vi "S4GUI.vi"() -> ()   [LabVIEW 2018] (continued)
            n1096 = call-dynamic "Write sequencia_ant.vi"("error in (no error)"=w2439, "sequencia_ant"=w2440, "Opt_Selector in"=w2442) -> ("error out"=w2438:errorcluster, "Opt_Selector out"=w2441:refnum<class "Opt_Selector.lvclass">)  [unwired: 7 in]
            n1097 = local write "P8"(w2447) -> ()
            n1098 = local write "P9"(w2447) -> ()
            n1099 = local write "P10"(w2447) -> ()
            n1100 = local write "P11"(w2447) -> ()
            n1101 = local write "P12"(w2445) -> ()
            n1102 = local write "P13"(w2445) -> ()
            n1103 = local write "P14"(w2445) -> ()
            n1104 = local write "P15"(w2445) -> ()
          }
          frame 1 {
            w2451 = u16 255 ("sequencia")
            w2458 = FALSE ("P0")
            w2459 = TRUE ("P0")
            w2460 = FALSE ("P0")
            w2461 = TRUE ("P0")
            # "0000 0000 1111 1111 = 255"
            n1105 = local write "P0"(w2461) -> ()
            n1106 = local write "P1"(w2461) -> ()
            n1107 = local write "P2"(w2461) -> ()
            n1108 = local write "P3"(w2461) -> ()
            n1109 = local write "P4"(w2459) -> ()
            n1110 = local write "P5"(w2459) -> ()
            n1111 = local write "P6"(w2459) -> ()
            n1112 = local write "P7"(w2459) -> ()
            n1113 = call-dynamic "Write sequencia.vi"("error in (no error)"=w2456, "sequencia"=w2451, "Opt_Selector in"=w2457) -> ("error out"=w2453:errorcluster, "Opt_Selector out"=w2455:refnum<class "Opt_Selector.lvclass">)  [unwired: 7 in]
            n1114 = local write "P8"(w2460) -> ()
            n1115 = local write "P9"(w2460) -> ()
            n1116 = local write "P10"(w2460) -> ()
            n1117 = local write "P11"(w2460) -> ()
            n1118 = local write "P12"(w2458) -> ()
            n1119 = local write "P13"(w2458) -> ()
            n1120 = local write "P14"(w2458) -> ()
            n1121 = local write "P15"(w2458) -> ()
            n1122 = call-dynamic "Write sequencia_ant.vi"("error in (no error)"=w2453, "sequencia_ant"=w2451, "Opt_Selector in"=w2455) -> ("error out"=w2452:errorcluster, "Opt_Selector out"=w2454:refnum<class "Opt_Selector.lvclass">)  [unwired: 7 in]
          }
          frame 2 {
            w2464 = u16 15 ("sequencia")
            w2471 = FALSE ("P0")
            w2472 = FALSE ("P0")
            w2473 = FALSE ("P0")
            w2474 = TRUE ("P0")
            # "0000 0000 0000 1111 = 15"
            n1123 = local write "P0"(w2474) -> ()
            n1124 = local write "P1"(w2474) -> ()
            n1125 = local write "P2"(w2474) -> ()
            n1126 = local write "P3"(w2474) -> ()
            n1127 = local write "P4"(w2472) -> ()
            n1128 = local write "P5"(w2472) -> ()
            n1129 = local write "P6"(w2472) -> ()
            n1130 = local write "P7"(w2472) -> ()
            n1131 = call-dynamic "Write sequencia.vi"("error in (no error)"=w2469, "sequencia"=w2464, "Opt_Selector in"=w2470) -> ("error out"=w2466:errorcluster, "Opt_Selector out"=w2468:refnum<class "Opt_Selector.lvclass">)  [unwired: 7 in]
            n1132 = call-dynamic "Write sequencia_ant.vi"("error in (no error)"=w2466, "sequencia_ant"=w2464, "Opt_Selector in"=w2468) -> ("error out"=w2465:errorcluster, "Opt_Selector out"=w2467:refnum<class "Opt_Selector.lvclass">)  [unwired: 7 in]
            n1133 = local write "P8"(w2473) -> ()
            n1134 = local write "P9"(w2473) -> ()
            n1135 = local write "P10"(w2473) -> ()
            n1136 = local write "P11"(w2473) -> ()
            n1137 = local write "P12"(w2471) -> ()
            n1138 = local write "P13"(w2471) -> ()
            n1139 = local write "P14"(w2471) -> ()
            n1140 = local write "P15"(w2471) -> ()
          }
          frame 3 {
            w2478 = u16 3855 ("sequencia")
            w2484 = FALSE ("P0")
            w2485 = FALSE ("P0")
            w2486 = TRUE ("P0")
            w2487 = TRUE ("P0")
            # "0000 1111 0000 1111 = 3855"
            n1141 = local write "P0"(w2487) -> ()
            n1142 = local write "P1"(w2487) -> ()
            n1143 = local write "P2"(w2487) -> ()
            n1144 = local write "P3"(w2487) -> ()
            n1145 = local write "P4"(w2485) -> ()
            n1146 = local write "P5"(w2485) -> ()
            n1147 = local write "P6"(w2485) -> ()
            n1148 = local write "P7"(w2485) -> ()
            n1149 = call-dynamic "Write sequencia.vi"("error in (no error)"=w2482, "sequencia"=w2478, "Opt_Selector in"=w2483) -> ("error out"=w2480:errorcluster, "Opt_Selector out"=w2481:refnum<class "Opt_Selector.lvclass">)  [unwired: 7 in]
            n1150 = local write "P8"(w2486) -> ()
            n1151 = local write "P9"(w2486) -> ()
            n1152 = local write "P10"(w2486) -> ()
            n1153 = local write "P11"(w2486) -> ()
            n1154 = local write "P12"(w2484) -> ()
            n1155 = local write "P13"(w2484) -> ()
            n1156 = local write "P14"(w2484) -> ()
            n1157 = local write "P15"(w2484) -> ()
            n1158 = call-dynamic "Write sequencia_ant.vi"("error in (no error)"=w2480, "sequencia_ant"=w2478, "Opt_Selector in"=w2481) -> ("error out"=w2479:errorcluster, "Opt_Selector out"=w2477:refnum<class "Opt_Selector.lvclass">)  [unwired: 7 in]
          }
          frame 4 {
            w2490 = u16 0 ("sequencia")
            w2497 = FALSE ("P0")
            w2498 = FALSE ("P0")
            w2499 = FALSE ("P0")
            w2500 = FALSE ("P0")
            n1159 = local write "P0"(w2500) -> ()
            n1160 = local write "P1"(w2500) -> ()
            n1161 = local write "P2"(w2500) -> ()
            n1162 = local write "P3"(w2500) -> ()
            n1163 = local write "P4"(w2498) -> ()
            n1164 = local write "P5"(w2498) -> ()
            n1165 = local write "P6"(w2498) -> ()
            n1166 = local write "P7"(w2498) -> ()
            n1167 = call-dynamic "Write sequencia.vi"("error in (no error)"=w2495, "sequencia"=w2490, "Opt_Selector in"=w2496) -> ("error out"=w2492:errorcluster, "Opt_Selector out"=w2494:refnum<class "Opt_Selector.lvclass">)  [unwired: 7 in]
            n1168 = call-dynamic "Write sequencia_ant.vi"("error in (no error)"=w2492, "sequencia_ant"=w2490, "Opt_Selector in"=w2494) -> ("error out"=w2491:errorcluster, "Opt_Selector out"=w2493:refnum<class "Opt_Selector.lvclass">)  [unwired: 7 in]
            n1169 = local write "P8"(w2499) -> ()
            n1170 = local write "P9"(w2499) -> ()
            n1171 = local write "P10"(w2499) -> ()
            n1172 = local write "P11"(w2499) -> ()
            n1173 = local write "P12"(w2497) -> ()
            n1174 = local write "P13"(w2497) -> ()
            n1175 = local write "P14"(w2497) -> ()
            n1176 = local write "P15"(w2497) -> ()
          }
          frame 5 {
          }
        }
        n1177 = call "Write WPROT.vi"("error in (no error)"=w2397, "Opt_Selector.lvclass"=w2404, "Instrument in"=w2403) -> ("error out"=w2406:errorcluster, "Instrument out"=w2407:refnum<class "Instrument.lvclass">)  [unwired: 7 in]
        n1178 = property on="#Polarimetric Sequence Done" class="Slide (strict)"(error in=w2397, "Scale.Maximum"=w2398, "Scale.Minimum"=w2396) -> ()  [unwired: 1 in, 2 out]
        n1179 = call "Write Instrument.lvclass.vi"("error in (no error)"=w2406, "Instrument.lvclass"=w2407, "S4ACS_GUI in"=w2402) -> ("error out"=w2386:errorcluster, "S4ACS_GUI out"=w2387:refnum<class "S4GUI.lvclass">)  [unwired: 7 in]
        n1180 = call "Read Instrument.lvclass.vi"("error in (no error)"=w2386, "S4ACS_GUI in"=w2387) -> ("error out"=w2391:errorcluster, "Instrument.lvclass"=w2392:refnum<class "Instrument.lvclass">, "S4ACS_GUI out"=w2395:refnum<class "S4GUI.lvclass">)  [unwired: 7 in]
        n1181 = call "Read ASEL.vi"("error in (no error)"=w2391, "Instrument in"=w2392) -> ("error out"=w2381:errorcluster, "Opt_Selector.lvclass"=w2383:refnum<class "Opt_Selector.lvclass">, "Instrument out"=w2388:refnum<class "Instrument.lvclass">)  [unwired: 7 in]
        n1182 = call "Read name_pos.vi"("error in (no error)"=w2381, "Optics in"=w2383) -> ("error out"=w2380:errorcluster, "name_pos"=w2379:string, "Optics out"=w2382:refnum<class "Opt_Selector.lvclass">)  [unwired: 7 in]
        n1183 = call "Write ASEL.vi"("error in (no error)"=w2380, "Opt_Selector.lvclass"=w2382, "Instrument in"=w2388) -> ("error out"=w2389:errorcluster, "Instrument out"=w2393:refnum<class "Instrument.lvclass">)  [unwired: 7 in]
        n1184 = case shown="\"ON\"" w2379 {
          tunnel: w2389 -> [w2412 w2423]
          tunnel: [w2412 w2419] -> w2390
          tunnel: w2393 -> [w2411 w2424]
          tunnel: [w2411 w2420] -> w2394
          frame Default {
          }
          frame "ON" {
            n1185 = call "Read WPROT.vi"("error in (no error)"=w2423, "Instrument in"=w2424) -> ("error out"=w2415:errorcluster, "Opt_Selector.lvclass"=w2422:refnum<class "Opt_Selector.lvclass">, "Instrument out"=w2421:refnum<class "Instrument.lvclass">)  [unwired: 7 in]
            n1186 = call-dynamic "Read sequencia.vi"("error in (no error)"=w2415, "Opt_Selector in"=w2422) -> ("error out"=w2414:errorcluster, "sequencia"=w2418:u16, "Opt_Selector out"=w2417:refnum<class "Opt_Selector.lvclass">)  [unwired: 7 in]
            n1187 = case shown="0" w2418 {
              tunnel: w2417 -> [w2426 w2435]
              tunnel: [w2426 w2431] -> w2416
              tunnel: w2414 -> [w2425 w2434]
              tunnel: [w2425 w2429] -> w2413
              frame Default {
              }
              frame 0 {
                n1188 = call-dynamic "Write sequencia.vi"("error in (no error)"=w2434, "sequencia"=u16 1, "Opt_Selector in"=w2435) -> ("error out"=w2430:errorcluster, "Opt_Selector out"=w2432:refnum<class "Opt_Selector.lvclass">)  [unwired: 7 in]
                n1189 = local write "P0"(TRUE ("P0")) -> ()
                n1190 = call-dynamic "Write sequencia_ant.vi"("error in (no error)"=w2430, "sequencia_ant"=u16 1, "Opt_Selector in"=w2432) -> ("error out"=w2429:errorcluster, "Opt_Selector out"=w2431:refnum<class "Opt_Selector.lvclass">)  [unwired: 7 in]
              }
            }
            n1191 = call "Write WPROT.vi"("error in (no error)"=w2413, "Opt_Selector.lvclass"=w2416, "Instrument in"=w2421) -> ("error out"=w2419:errorcluster, "Instrument out"=w2420:refnum<class "Instrument.lvclass">)  [unwired: 7 in]
          }
        }
        n1192 = call "Write Instrument.lvclass.vi"("error in (no error)"=w2390, "Instrument.lvclass"=w2394, "S4ACS_GUI in"=w2395) -> ("error out"=w2385:errorcluster, "S4ACS_GUI out"=w2384:refnum<class "S4GUI.lvclass">)  [unwired: 7 in]
      }
      event "P0", "P1", "P2", "P3", "P4", "P5", "P6", "P7", "P8", "P9", "P10", "P11", "P12", "P13", "P14", "P15": Value Change {
        w2558 = u16 5 items=["All 16 positions", "First 8 positions", "First 4 positions", "0-3 + 8-11", "Clear", "Customized"] ("Select Positions")
        # "Garantir que, quando em POLARIMETRIA, pelo menos WP1 esteja selecionado."
        # "Salva tambem em \nSequencia_ant para\no caso de repeticao."
        n1193 = event-data() -> ()  [unwired: 1 in, 6 out]
        n1194 = local write "Select Positions"(w2558) -> ()
        n1195 = call "Read Instrument.lvclass.vi"("error in (no error)"=w2540, "S4ACS_GUI in"=w2541) -> ("error out"=w2535:errorcluster, "Instrument.lvclass"=w2538:refnum<class "Instrument.lvclass">, "S4ACS_GUI out"=w2539:refnum<class "S4GUI.lvclass">)  [unwired: 7 in]
        n1196 = Build Array("P0", "P1", "P2", "P3", "P4", "P5", "P6", "P7", "P8", "P9", "P10", "P11", "P12", "P13", "P14", "P15") -> (w2526:bool[])
        n1197 = call "Read WPROT.vi"("error in (no error)"=w2535, "Instrument in"=w2538) -> ("error out"=w2534:errorcluster, "Opt_Selector.lvclass"=w2536:refnum<class "Opt_Selector.lvclass">, "Instrument out"=w2537:refnum<class "Instrument.lvclass">)  [unwired: 7 in]
        n1198 = Boolean Array To Number(Boolean array=w2526) -> (number=w2542:u32)
        n1199 = To Unsigned Word Integer(number=w2542) -> (unsigned 16bit integer=w2527:u16)
        n1200 = call-dynamic "Write sequencia.vi"("error in (no error)"=w2534, "sequencia"=w2527, "Opt_Selector in"=w2536) -> ("error out"=w2529:errorcluster, "Opt_Selector out"=w2531:refnum<class "Opt_Selector.lvclass">)  [unwired: 7 in]
        n1201 = call-dynamic "Write sequencia_ant.vi"("error in (no error)"=w2529, "sequencia_ant"=w2527, "Opt_Selector in"=w2531) -> ("error out"=w2528:errorcluster, "Opt_Selector out"=w2530:refnum<class "Opt_Selector.lvclass">)  [unwired: 7 in]
        n1202 = for {
          tunnel: w2526 -> [w2587] mode=indexing
          shift-right: [w2586] -> w2524
          shift-left: 0 -> [w2584]
          # "calcula qtd de 1s"
          n1203 = Increment(x=w2584) -> (x+1=w2585:i32)
          n1204 = Select(t=w2585, s=w2587, f=w2584) -> (s? t:f=w2586:i32)
        }
        n1205 = call "Write WPROT.vi"("error in (no error)"=w2528, "Opt_Selector.lvclass"=w2530, "Instrument in"=w2537) -> ("error out"=w2533:errorcluster, "Instrument out"=w2532:refnum<class "Instrument.lvclass">)  [unwired: 7 in]
        n1206 = call "Write Instrument.lvclass.vi"("error in (no error)"=w2533, "Instrument.lvclass"=w2532, "S4ACS_GUI in"=w2539) -> ("error out"=w2507:errorcluster, "S4ACS_GUI out"=w2508:refnum<class "S4GUI.lvclass">)  [unwired: 7 in]
        n1207 = property on="#Polarimetric Sequence Done" class="Slide (strict)"("Scale.Maximum"=w2524, "Scale.Minimum"=0.0 ("Scale.Range:Minimum")) -> ()  [unwired: 2 in, 2 out]
        n1208 = call "Read Instrument.lvclass.vi"("error in (no error)"=w2507, "S4ACS_GUI in"=w2508) -> ("error out"=w2513:errorcluster, "Instrument.lvclass"=w2512:refnum<class "Instrument.lvclass">, "S4ACS_GUI out"=w2509:refnum<class "S4GUI.lvclass">)  [unwired: 7 in]
        n1209 = call "Read ASEL.vi"("error in (no error)"=w2513, "Instrument in"=w2512) -> ("error out"=w2519:errorcluster, "Opt_Selector.lvclass"=w2517:refnum<class "Opt_Selector.lvclass">, "Instrument out"=w2516:refnum<class "Instrument.lvclass">)  [unwired: 7 in]
        n1210 = call "Read name_pos.vi"("error in (no error)"=w2519, "Optics in"=w2517) -> ("error out"=w2520:errorcluster, "name_pos"=w2521:string, "Optics out"=w2518:refnum<class "Opt_Selector.lvclass">)  [unwired: 7 in]
        n1211 = call "Write ASEL.vi"("error in (no error)"=w2520, "Opt_Selector.lvclass"=w2518, "Instrument in"=w2516) -> ("error out"=w2515:errorcluster, "Instrument out"=w2511:refnum<class "Instrument.lvclass">)  [unwired: 7 in]
        n1212 = case shown="\"ON\"" w2521 {
          tunnel: w2515 -> [w2560 w2571]
          tunnel: [w2560 w2567] -> w2514
          tunnel: w2511 -> [w2559 w2572]
          tunnel: [w2559 w2568] -> w2510
          frame Default {
          }
          frame "ON" {
            n1213 = call "Read WPROT.vi"("error in (no error)"=w2571, "Instrument in"=w2572) -> ("error out"=w2563:errorcluster, "Opt_Selector.lvclass"=w2570:refnum<class "Opt_Selector.lvclass">, "Instrument out"=w2569:refnum<class "Instrument.lvclass">)  [unwired: 7 in]
            n1214 = call-dynamic "Read sequencia.vi"("error in (no error)"=w2563, "Opt_Selector in"=w2570) -> ("error out"=w2562:errorcluster, "sequencia"=w2566:u16, "Opt_Selector out"=w2565:refnum<class "Opt_Selector.lvclass">)  [unwired: 7 in]
            n1215 = case shown="0" w2566 {
              tunnel: w2565 -> [w2574 w2583]
              tunnel: [w2574 w2579] -> w2564
              tunnel: w2562 -> [w2573 w2582]
              tunnel: [w2573 w2577] -> w2561
              frame Default {
              }
              frame 0 {
                n1216 = call-dynamic "Write sequencia.vi"("error in (no error)"=w2582, "sequencia"=u16 1, "Opt_Selector in"=w2583) -> ("error out"=w2578:errorcluster, "Opt_Selector out"=w2580:refnum<class "Opt_Selector.lvclass">)  [unwired: 7 in]
                n1217 = local write "P0"(TRUE ("P0")) -> ()
                n1218 = call-dynamic "Write sequencia_ant.vi"("error in (no error)"=w2578, "sequencia_ant"=u16 1, "Opt_Selector in"=w2580) -> ("error out"=w2577:errorcluster, "Opt_Selector out"=w2579:refnum<class "Opt_Selector.lvclass">)  [unwired: 7 in]
              }
            }
            n1219 = call "Write WPROT.vi"("error in (no error)"=w2561, "Opt_Selector.lvclass"=w2564, "Instrument in"=w2569) -> ("error out"=w2567:errorcluster, "Instrument out"=w2568:refnum<class "Instrument.lvclass">)  [unwired: 7 in]
          }
        }
        n1220 = call "Write Instrument.lvclass.vi"("error in (no error)"=w2514, "Instrument.lvclass"=w2510, "S4ACS_GUI in"=w2509) -> ("error out"=w2505:errorcluster, "S4ACS_GUI out"=w2506:refnum<class "S4GUI.lvclass">)  [unwired: 7 in]
      }
      event "SSM": Value Change {
        # "F: fotom.\nT: polar."
        n1221 = event-data() -> ()  [unwired: 1 in, 6 out]
        n1222 = call-dynamic "Read mode EXPOSE.vi"("error in (no error)"=w2593, "S4GUI in"=w2594) -> ("error out"=w2592:errorcluster, "mode EXPOSE"=w2588:bool, "S4GUI out"=w2589:refnum<class "S4GUI.lvclass">)  [unwired: 7 in]
        n1223 = call "Read Instrument.lvclass.vi"("error in (no error)"=w2592, "S4ACS_GUI in"=w2589) -> ("error out"=w2591:errorcluster, "Instrument.lvclass"=w2597:refnum<class "Instrument.lvclass">, "S4ACS_GUI out"=w2596:refnum<class "S4GUI.lvclass">)  [unwired: 7 in]
        n1224 = call-dynamic "Read mode.vi"("error in (no error)"=w2591, "Instrument in"=w2597) -> ("error out"=w2590:errorcluster, "mode"=w2595:bool)  [unwired: 7 in, 1 out]
        n1225 = case shown="0, Default" "SSM" {
          tunnel: [T7."Enabled" ("Disabled") T7."Disabled and Grayed Out" ("Disabled")] -> w2630
          tunnel: [T7."Disabled and Grayed Out" ("Disabled") T7."Enabled" ("Disabled")] -> w2611
          tunnel: [w2646 "Start" ("Caption.Text")] -> w2622
          tunnel: [w2646 "Stop" ("Caption.Text")] -> w2615
          tunnel: [w2646 "Abort" ("Caption.Text")] -> w2610
          tunnel: [w2646 "Pause" ("Caption.Text")] -> w2617
          tunnel: [TRUE FALSE] -> w2628
          tunnel: [T7."Enabled" ("Disabled") T7."Disabled and Grayed Out" ("Disabled")] -> w2625
          tunnel: [T7."Disabled and Grayed Out" ("Disabled") T7."Enabled" ("Disabled")] -> w2605
          tunnel: w2590 -> [w2638 w2873]
          tunnel: w2596 -> [w2640 w2872]
          tunnel: [w2642 w2864] -> w2603
          tunnel: [w2634 w2863] -> w2602
          tunnel: w2595 -> [_ w2849]
          tunnel: w2588 -> [_ w2847]
          frame 1 {
            w2646 = "Sync" ("Caption.Text")
            # "Sync mode: Os canais sao configurados para Trigger externo, desde que o SyncBox esteja conectado."
            # "Sync by Cycle"
            n1226 = call-dynamic "Read Sync Box.lvclass.vi"("error in (no error)"=w2638, "SPARC4_AC in"=w2640) -> ("error out"=w2637:errorcluster, "Sync Box.lvclass"=w2641:refnum<class "Sync Box.lvclass">, "SPARC4_AC out"=w2639:refnum<class "S4GUI.lvclass">)  [unwired: 7 in]
            n1227 = call "Read connection.vi"("error in (no error)"=w2637, "Server in"=w2641) -> ("error out"=w2636:errorcluster, "connection"=w2635:bool)  [unwired: 7 in, 1 out]
            n1228 = case shown="True" w2635 {
              tunnel: [w2650 w2667] -> w2642
              tunnel: w2639 -> [w2650 w2657]
              tunnel: w2636 -> [w2649 w2656]
              tunnel: [w2649 w2651] -> w2634
              frame False {
              }
              frame True {
                n1229 = call-dynamic "Read AcquisitionC.vi"("error in (no error)"=w2656, "S4ACS_GUI in"=w2657) -> ("error out"=w2674:errorcluster, "Acquisition.lvclass"=w2673:refnum<class "Acquisition.lvclass">)  [unwired: 7 in, 1 out]
                n1230 = call-dynamic "Read AcquisitionA.vi"("error in (no error)"=w2656, "S4ACS_GUI in"=w2657) -> ("error out"=w2677:errorcluster, "Acquisition.lvclass"=w2678:refnum<class "Acquisition.lvclass">, "S4ACS_GUI out"=w2666:refnum<class "S4GUI.lvclass">)  [unwired: 7 in]
                n1231 = call "Read AcquisitionB.vi"("error in (no error)"=w2656, "S4ACS_GUI in"=w2657) -> ("error out"=w2675:errorcluster, "Acquisition.lvclass"=w2676:refnum<class "Acquisition.lvclass">)  [unwired: 7 in, 1 out]
                n1232 = call-dynamic "Read AcquisitionD.vi"("error in (no error)"=w2656, "S4ACS_GUI in"=w2657) -> ("error out"=w2671:errorcluster, "Acquisition.lvclass"=w2672:refnum<class "Acquisition.lvclass">)  [unwired: 7 in, 1 out]
                n1233 = call "Read connection.vi"("error in (no error)"=w2671, "Server in"=w2672) -> ("error out"=w2680:errorcluster, "connection"=w2679:bool, "Server out"=w2681:refnum<class "Acquisition.lvclass">)  [unwired: 7 in]
                n1234 = call "Read connection.vi"("error in (no error)"=w2674, "Server in"=w2673) -> ("error out"=w2683:errorcluster, "connection"=w2682:bool, "Server out"=w2684:refnum<class "Acquisition.lvclass">)  [unwired: 7 in]
                n1235 = call "Read connection.vi"("error in (no error)"=w2675, "Server in"=w2676) -> ("error out"=w2686:errorcluster, "connection"=w2685:bool, "Server out"=w2687:refnum<class "Acquisition.lvclass">)  [unwired: 7 in]
                n1236 = call "Read connection.vi"("error in (no error)"=w2677, "Server in"=w2678) -> ("error out"=w2689:errorcluster, "connection"=w2688:bool, "Server out"=w2690:refnum<class "Acquisition.lvclass">)  [unwired: 7 in]
                n1237 = case shown="True" w2685 {
                  tunnel: w2687 -> [w2770 w2774]
                  tunnel: w2686 -> [w2769 w2773]
                  tunnel: [w2770 w2772] -> w2663
                  tunnel: [w2769 w2771] -> w2662
                  frame False {
                  }
                  frame True {
                    # "Ext Start"
                    # "nome do arquivo .cfg"
                    # "seção no arquivo .cfg"
                    n1238 = call-dynamic "Read Channel.vi"("error in (no error)"=w2773, "Acquisition in"=w2774) -> ("error out"=w2778:errorcluster, "Channel.lvclass"=w2777:refnum<class "Channel.lvclass">, "Acquisition out"=w2776:refnum<class "Acquisition.lvclass">)  [unwired: 7 in]
                    n1239 = call-dynamic "Read Interface.vi"("error in (no error)"=w2778, "Channel in"=w2777) -> ("error out"=w2786:errorcluster, "Interface.lvclass"=w2787:refnum<class "Interface.lvclass">, "Channel out"=w2775:refnum<class "Channel.lvclass">)  [unwired: 7 in]
                    n1240 = call-dynamic "Get CCD_Config.vi"("error in (no error)"=w2786, "Interface in"=w2787) -> ("error out"=w2783:errorcluster, "output cluster"=w2782:T24, "Interface out"=w2788:refnum<class "Interface.lvclass">)  [unwired: 7 in]
                    n1241 = Bundle By Name(cluster=w2782, "TRIGGER_MODE"=u8 6 ("SHUTTER_MODE")) -> (w2784:T24)
                    n1242 = call-dynamic "Set CCD_Config.vi"("error in (no error)"=w2783, "input cluster"=w2784, "Interface in"=w2788) -> ("error out"=w2781:errorcluster, "Interface out"=w2789:refnum<class "Interface.lvclass">)  [unwired: 7 in]
                    n1243 = Flatten To String(anything=w2784, error in (no error)=w2781) -> (data string=w2779:string, error out=w2780:errorcluster)  [unwired: 2 in, 1 out]
                    n1244 = call "Write flatted cluster.vi"("error in (no error)"=w2780, "flatted cluster"=w2779, "Interface in"=w2789) -> ("error out"=w2791:errorcluster, "Interface out"=w2790:refnum<class "Interface.lvclass">)  [unwired: 7 in]
                    n1245 = call-dynamic "Write Interface.vi"("error in (no error)"=w2791, "Interface.lvclass"=w2790, "Channel in"=w2775) -> ("error out"=w2797:errorcluster, "Channel out"=w2798:refnum<class "Channel.lvclass">)  [unwired: 7 in]
                    n1246 = call "Write section_name.vi"("error in (no error)"=w2797, "section_name"="CCD_ACS2", "Channel in"=w2798) -> ("error out"=w2795:errorcluster, "Channel out"=w2801:refnum<class "Channel.lvclass">)  [unwired: 7 in]
                    n1247 = call-dynamic "save config.vi"("error in (no error)"=w2795, "file config"="lastsaved.cfg", "Channel in"=w2801) -> ("error out"=w2796:errorcluster, "Channel out"=w2802:refnum<class "Channel.lvclass">)  [unwired: 7 in]
                    n1248 = call-dynamic "Read State Machine.vi"("error in (no error)"=w2796, "Device in"=w2802) -> ("error out"=w2792:errorcluster, "State Machine.lvclass"=w2804:refnum<class "State Machine.lvclass">, "Device out"=w2803:refnum<class "Channel.lvclass">)  [unwired: 7 in]
                    n1249 = call-dynamic "Write State.vi"("error in (no error)"=w2792, "State"=60, "State Machine in"=w2804) -> ("error out"=w2793:errorcluster, "State Machine out"=w2805:refnum<class "State Machine.lvclass">)  [unwired: 7 in]
                    n1250 = call-dynamic "Write State Machine.vi"("error in (no error)"=w2793, "State Machine.lvclass"=w2805, "Device in"=w2803) -> ("error out"=w2807:errorcluster, "Device out"=w2806:refnum<class "Channel.lvclass">)  [unwired: 7 in]
                    n1251 = call-dynamic "Write Channel.vi"("error in (no error)"=w2807, "Channel.lvclass"=w2806, "Acquisition in"=w2776) -> ("error out"=w2771:errorcluster, "Acquisition out"=w2772:refnum<class "Acquisition.lvclass">)  [unwired: 7 in]
                  }
                }
                n1252 = case shown="True" w2688 {
                  tunnel: [w2808 w2842] -> w2664
                  tunnel: [w2809 w2841] -> w2665
                  tunnel: w2690 -> [w2809 w2811]
                  tunnel: w2689 -> [w2808 w2810]
                  frame False {
                  }
                  frame True {
                    # "nome do arquivo .cfg"
                    # "seção no arquivo .cfg"
                    # "Ext Start"
                    n1253 = call-dynamic "Read Channel.vi"("error in (no error)"=w2810, "Acquisition in"=w2811) -> ("error out"=w2843:errorcluster, "Channel.lvclass"=w2844:refnum<class "Channel.lvclass">, "Acquisition out"=w2845:refnum<class "Acquisition.lvclass">)  [unwired: 7 in]
                    n1254 = call-dynamic "Read Interface.vi"("error in (no error)"=w2843, "Channel in"=w2844) -> ("error out"=w2833:errorcluster, "Interface.lvclass"=w2832:refnum<class "Interface.lvclass">, "Channel out"=w2846:refnum<class "Channel.lvclass">)  [unwired: 7 in]
                    n1255 = call-dynamic "Get CCD_Config.vi"("error in (no error)"=w2833, "Interface in"=w2832) -> ("error out"=w2836:errorcluster, "output cluster"=w2837:T24, "Interface out"=w2831:refnum<class "Interface.lvclass">)  [unwired: 7 in]
                    n1256 = Bundle By Name(cluster=w2837, "TRIGGER_MODE"=u8 6 ("SHUTTER_MODE")) -> (w2835:T24)
                    n1257 = call-dynamic "Set CCD_Config.vi"("error in (no error)"=w2836, "input cluster"=w2835, "Interface in"=w2831) -> ("error out"=w2838:errorcluster, "Interface out"=w2830:refnum<class "Interface.lvclass">)  [unwired: 7 in]
                    n1258 = Flatten To String(anything=w2835, error in (no error)=w2838) -> (data string=w2840:string, error out=w2839:errorcluster)  [unwired: 2 in, 1 out]
                    n1259 = call "Write flatted cluster.vi"("error in (no error)"=w2839, "flatted cluster"=w2840, "Interface in"=w2830) -> ("error out"=w2828:errorcluster, "Interface out"=w2829:refnum<class "Interface.lvclass">)  [unwired: 7 in]
                    n1260 = call-dynamic "Write Interface.vi"("error in (no error)"=w2828, "Interface.lvclass"=w2829, "Channel in"=w2846) -> ("error out"=w2823:errorcluster, "Channel out"=w2822:refnum<class "Channel.lvclass">)  [unwired: 7 in]
                    n1261 = call "Write section_name.vi"("error in (no error)"=w2823, "section_name"="CCD_ACS1", "Channel in"=w2822) -> ("error out"=w2824:errorcluster, "Channel out"=w2819:refnum<class "Channel.lvclass">)  [unwired: 7 in]
                    n1262 = call-dynamic "save config.vi"("error in (no error)"=w2824, "file config"="lastsaved.cfg", "Channel in"=w2819) -> ("error out"=w2812:errorcluster, "Channel out"=w2813:refnum<class "Channel.lvclass">)  [unwired: 7 in]
                    n1263 = call-dynamic "Read State Machine.vi"("error in (no error)"=w2812, "Device in"=w2813) -> ("error out"=w2827:errorcluster, "State Machine.lvclass"=w2817:refnum<class "State Machine.lvclass">, "Device out"=w2818:refnum<class "Channel.lvclass">)  [unwired: 7 in]
                    n1264 = call-dynamic "Write State.vi"("error in (no error)"=w2827, "State"=60, "State Machine in"=w2817) -> ("error out"=w2826:errorcluster, "State Machine out"=w2816:refnum<class "State Machine.lvclass">)  [unwired: 7 in]
                    n1265 = call-dynamic "Write State Machine.vi"("error in (no error)"=w2826, "State Machine.lvclass"=w2816, "Device in"=w2818) -> ("error out"=w2814:errorcluster, "Device out"=w2815:refnum<class "Channel.lvclass">)  [unwired: 7 in]
                    n1266 = call-dynamic "Write Channel.vi"("error in (no error)"=w2814, "Channel.lvclass"=w2815, "Acquisition in"=w2845) -> ("error out"=w2842:errorcluster, "Acquisition out"=w2841:refnum<class "Acquisition.lvclass">)  [unwired: 7 in]
                  }
                }
                n1267 = case shown="True" w2682 {
                  tunnel: w2684 -> [w2731 w2735]
                  tunnel: w2683 -> [w2730 w2734]
                  tunnel: [w2731 w2733] -> w2661
                  tunnel: [w2730 w2732] -> w2660
                  frame False {
                  }
                  frame True {
                    # "Ext Start"
                    # "nome do arquivo .cfg"
                    # "seção no arquivo .cfg"
                    n1268 = call-dynamic "Read Channel.vi"("error in (no error)"=w2734, "Acquisition in"=w2735) -> ("error out"=w2739:errorcluster, "Channel.lvclass"=w2738:refnum<class "Channel.lvclass">, "Acquisition out"=w2737:refnum<class "Acquisition.lvclass">)  [unwired: 7 in]
                    n1269 = call-dynamic "Read Interface.vi"("error in (no error)"=w2739, "Channel in"=w2738) -> ("error out"=w2747:errorcluster, "Interface.lvclass"=w2748:refnum<class "Interface.lvclass">, "Channel out"=w2736:refnum<class "Channel.lvclass">)  [unwired: 7 in]
                    n1270 = call-dynamic "Get CCD_Config.vi"("error in (no error)"=w2747, "Interface in"=w2748) -> ("error out"=w2744:errorcluster, "output cluster"=w2743:T24, "Interface out"=w2749:refnum<class "Interface.lvclass">)  [unwired: 7 in]
                    n1271 = Bundle By Name(cluster=w2743, "TRIGGER_MODE"=u8 6 ("SHUTTER_MODE")) -> (w2745:T24)
                    n1272 = call-dynamic "Set CCD_Config.vi"("error in (no error)"=w2744, "input cluster"=w2745, "Interface in"=w2749) -> ("error out"=w2742:errorcluster, "Interface out"=w2750:refnum<class "Interface.lvclass">)  [unwired: 7 in]
                    n1273 = Flatten To String(anything=w2745, error in (no error)=w2742) -> (data string=w2740:string, error out=w2741:errorcluster)  [unwired: 2 in, 1 out]
                    n1274 = call "Write flatted cluster.vi"("error in (no error)"=w2741, "flatted cluster"=w2740, "Interface in"=w2750) -> ("error out"=w2752:errorcluster, "Interface out"=w2751:refnum<class "Interface.lvclass">)  [unwired: 7 in]
                    n1275 = call-dynamic "Write Interface.vi"("error in (no error)"=w2752, "Interface.lvclass"=w2751, "Channel in"=w2736) -> ("error out"=w2758:errorcluster, "Channel out"=w2759:refnum<class "Channel.lvclass">)  [unwired: 7 in]
                    n1276 = call "Write section_name.vi"("error in (no error)"=w2758, "section_name"="CCD_ACS3", "Channel in"=w2759) -> ("error out"=w2756:errorcluster, "Channel out"=w2762:refnum<class "Channel.lvclass">)  [unwired: 7 in]
                    n1277 = call-dynamic "save config.vi"("error in (no error)"=w2756, "file config"="lastsaved.cfg", "Channel in"=w2762) -> ("error out"=w2757:errorcluster, "Channel out"=w2763:refnum<class "Channel.lvclass">)  [unwired: 7 in]
                    n1278 = call-dynamic "Read State Machine.vi"("error in (no error)"=w2757, "Device in"=w2763) -> ("error out"=w2753:errorcluster, "State Machine.lvclass"=w2765:refnum<class "State Machine.lvclass">, "Device out"=w2764:refnum<class "Channel.lvclass">)  [unwired: 7 in]
                    n1279 = call-dynamic "Write State.vi"("error in (no error)"=w2753, "State"=60, "State Machine in"=w2765) -> ("error out"=w2754:errorcluster, "State Machine out"=w2766:refnum<class "State Machine.lvclass">)  [unwired: 7 in]
                    n1280 = call-dynamic "Write State Machine.vi"("error in (no error)"=w2754, "State Machine.lvclass"=w2766, "Device in"=w2764) -> ("error out"=w2768:errorcluster, "Device out"=w2767:refnum<class "Channel.lvclass">)  [unwired: 7 in]
                    n1281 = call-dynamic "Write Channel.vi"("error in (no error)"=w2768, "Channel.lvclass"=w2767, "Acquisition in"=w2737) -> ("error out"=w2732:errorcluster, "Acquisition out"=w2733:refnum<class "Acquisition.lvclass">)  [unwired: 7 in]
                  }
                }
                n1282 = case shown="True" w2679 {
                  tunnel: w2681 -> [w2692 w2696]
                  tunnel: w2680 -> [w2691 w2695]
                  tunnel: [w2692 w2694] -> w2659
                  tunnel: [w2691 w2693] -> w2658
                  frame False {
                  }
                  frame True {
                    # "Ext Start"
                    # "nome do arquivo .cfg"
                    # "seção no arquivo .cfg"
                    n1283 = call-dynamic "Read Channel.vi"("error in (no error)"=w2695, "Acquisition in"=w2696) -> ("error out"=w2726:errorcluster, "Channel.lvclass"=w2727:refnum<class "Channel.lvclass">, "Acquisition out"=w2728:refnum<class "Acquisition.lvclass">)  [unwired: 7 in]
                    n1284 = call-dynamic "Read Interface.vi"("error in (no error)"=w2726, "Channel in"=w2727) -> ("error out"=w2718:errorcluster, "Interface.lvclass"=w2717:refnum<class "Interface.lvclass">, "Channel out"=w2729:refnum<class "Channel.lvclass">)  [unwired: 7 in]
                    n1285 = call-dynamic "Get CCD_Config.vi"("error in (no error)"=w2718, "Interface in"=w2717) -> ("error out"=w2721:errorcluster, "output cluster"=w2722:T24, "Interface out"=w2716:refnum<class "Interface.lvclass">)  [unwired: 7 in]
                    n1286 = Bundle By Name(cluster=w2722, "TRIGGER_MODE"=u8 6 ("SHUTTER_MODE")) -> (w2720:T24)
                    n1287 = call-dynamic "Set CCD_Config.vi"("error in (no error)"=w2721, "input cluster"=w2720, "Interface in"=w2716) -> ("error out"=w2723:errorcluster, "Interface out"=w2715:refnum<class "Interface.lvclass">)  [unwired: 7 in]
                    n1288 = Flatten To String(anything=w2720, error in (no error)=w2723) -> (data string=w2725:string, error out=w2724:errorcluster)  [unwired: 2 in, 1 out]
                    n1289 = call "Write flatted cluster.vi"("error in (no error)"=w2724, "flatted cluster"=w2725, "Interface in"=w2715) -> ("error out"=w2713:errorcluster, "Interface out"=w2714:refnum<class "Interface.lvclass">)  [unwired: 7 in]
                    n1290 = call-dynamic "Write Interface.vi"("error in (no error)"=w2713, "Interface.lvclass"=w2714, "Channel in"=w2729) -> ("error out"=w2707:errorcluster, "Channel out"=w2706:refnum<class "Channel.lvclass">)  [unwired: 7 in]
                    n1291 = call "Write section_name.vi"("error in (no error)"=w2707, "section_name"="CCD_ACS4", "Channel in"=w2706) -> ("error out"=w2709:errorcluster, "Channel out"=w2703:refnum<class "Channel.lvclass">)  [unwired: 7 in]
                    n1292 = call-dynamic "save config.vi"("error in (no error)"=w2709, "file config"="lastsaved.cfg", "Channel in"=w2703) -> ("error out"=w2708:errorcluster, "Channel out"=w2702:refnum<class "Channel.lvclass">)  [unwired: 7 in]
                    n1293 = call-dynamic "Read State Machine.vi"("error in (no error)"=w2708, "Device in"=w2702) -> ("error out"=w2712:errorcluster, "State Machine.lvclass"=w2700:refnum<class "State Machine.lvclass">, "Device out"=w2701:refnum<class "Channel.lvclass">)  [unwired: 7 in]
                    n1294 = call-dynamic "Write State.vi"("error in (no error)"=w2712, "State"=60, "State Machine in"=w2700) -> ("error out"=w2711:errorcluster, "State Machine out"=w2699:refnum<class "State Machine.lvclass">)  [unwired: 7 in]
                    n1295 = call-dynamic "Write State Machine.vi"("error in (no error)"=w2711, "State Machine.lvclass"=w2699, "Device in"=w2701) -> ("error out"=w2697:errorcluster, "Device out"=w2698:refnum<class "Channel.lvclass">)  [unwired: 7 in]
                    n1296 = call-dynamic "Write Channel.vi"("error in (no error)"=w2697, "Channel.lvclass"=w2698, "Acquisition in"=w2728) -> ("error out"=w2693:errorcluster, "Acquisition out"=w2694:refnum<class "Acquisition.lvclass">)  [unwired: 7 in]
                  }
                }
                n1297 = call-dynamic "Write AcquisitionA.vi"("error in (no error)"=w2664, "Acquisition.lvclass"=w2665, "S4ACS_GUI in"=w2666) -> ("error out"=w2655:errorcluster, "S4ACS_GUI out"=w2670:refnum<class "S4GUI.lvclass">)  [unwired: 7 in]
                n1298 = call "Write AcquisitionB.vi"("error in (no error)"=w2662, "Acquisition.lvclass"=w2663, "S4ACS_GUI in"=w2670) -> ("error out"=w2654:errorcluster, "S4ACS_GUI out"=w2669:refnum<class "S4GUI.lvclass">)  [unwired: 7 in]
                n1299 = call-dynamic "Write AcquisitionC.vi"("error in (no error)"=w2660, "Acquisition.lvclass"=w2661, "S4ACS_GUI in"=w2669) -> ("error out"=w2653:errorcluster, "S4ACS_GUI out"=w2668:refnum<class "S4GUI.lvclass">)  [unwired: 7 in]
                n1300 = call-dynamic "Write AcquisitionD.vi"("error in (no error)"=w2658, "Acquisition.lvclass"=w2659, "S4ACS_GUI in"=w2668) -> ("error out"=w2652:errorcluster, "S4ACS_GUI out"=w2667:refnum<class "S4GUI.lvclass">)  [unwired: 7 in]
                n1301 = Merge Errors(w2655, w2654, w2653, w2652) -> (w2651:errorcluster)
              }
            }
          }
          frame 0, Default {
            # "Async mode: Os canais são configurados com Trigger Interno para Fotometria ou Trigger Externo para Polarimetria (independentemente do status do SyncBox)"
            # "Aynchronous:"
            n1302 = call-dynamic "Read AcquisitionC.vi"("error in (no error)"=w2873, "S4ACS_GUI in"=w2872) -> ("error out"=w2877:errorcluster, "Acquisition.lvclass"=w2876:refnum<class "Acquisition.lvclass">)  [unwired: 7 in, 1 out]
            n1303 = call "Read AcquisitionB.vi"("error in (no error)"=w2873, "S4ACS_GUI in"=w2872) -> ("error out"=w2878:errorcluster, "Acquisition.lvclass"=w2879:refnum<class "Acquisition.lvclass">)  [unwired: 7 in, 1 out]
            n1304 = call-dynamic "Read AcquisitionA.vi"("error in (no error)"=w2873, "S4ACS_GUI in"=w2872) -> ("error out"=w2880:errorcluster, "Acquisition.lvclass"=w2881:refnum<class "Acquisition.lvclass">, "S4ACS_GUI out"=w2862:refnum<class "S4GUI.lvclass">)  [unwired: 7 in]
            n1305 = case shown="True" w2849 {
              tunnel: [u8 0 ("SHUTTER_MODE") w2900] -> w2848
              tunnel: w2847 -> [_ w2903]
              frame False {
                # "Fotom."
                # "Internal"
              }
              frame True {
                # "exp mode?"
                # "Internal"
                # "Polar."
                # "Ext. Start"
                n1306 = Select(t=u8 0, s=w2903, f=u8 6 ("SHUTTER_MODE")) -> (s? t:f=w2900:u8)
              }
            }
            n1307 = call-dynamic "Read AcquisitionD.vi"("error in (no error)"=w2873, "S4ACS_GUI in"=w2872) -> ("error out"=w2874:errorcluster, "Acquisition.lvclass"=w2875:refnum<class "Acquisition.lvclass">)  [unwired: 7 in, 1 out]
            n1308 = call "Read connection.vi"("error in (no error)"=w2877, "Server in"=w2876) -> ("error out"=w2886:errorcluster, "connection"=w2885:bool, "Server out"=w2887:refnum<class "Acquisition.lvclass">)  [unwired: 7 in]
            n1309 = call "Read connection.vi"("error in (no error)"=w2878, "Server in"=w2879) -> ("error out"=w2889:errorcluster, "connection"=w2888:bool, "Server out"=w2890:refnum<class "Acquisition.lvclass">)  [unwired: 7 in]
            n1310 = call "Read connection.vi"("error in (no error)"=w2874, "Server in"=w2875) -> ("error out"=w2883:errorcluster, "connection"=w2882:bool, "Server out"=w2884:refnum<class "Acquisition.lvclass">)  [unwired: 7 in]
            n1311 = call "Read connection.vi"("error in (no error)"=w2880, "Server in"=w2881) -> ("error out"=w2892:errorcluster, "connection"=w2891:bool, "Server out"=w2893:refnum<class "Acquisition.lvclass">)  [unwired: 7 in]
            n1312 = case shown="True" w2885 {
              tunnel: w2887 -> [w2944 w2949]
              tunnel: w2886 -> [w2943 w2948]
              tunnel: [w2944 w2947] -> w2857
              tunnel: [w2943 w2946] -> w2856
              tunnel: w2848 -> [_ w2945]
              frame False {
              }
              frame True {
                # "nome do arquivo .cfg"
                # "seção no arquivo .cfg"
                n1313 = call-dynamic "Read Channel.vi"("error in (no error)"=w2948, "Acquisition in"=w2949) -> ("error out"=w2953:errorcluster, "Channel.lvclass"=w2952:refnum<class "Channel.lvclass">, "Acquisition out"=w2951:refnum<class "Acquisition.lvclass">)  [unwired: 7 in]
                n1314 = call-dynamic "Read Interface.vi"("error in (no error)"=w2953, "Channel in"=w2952) -> ("error out"=w2960:errorcluster, "Interface.lvclass"=w2961:refnum<class "Interface.lvclass">, "Channel out"=w2950:refnum<class "Channel.lvclass">)  [unwired: 7 in]
                n1315 = call-dynamic "Get CCD_Config.vi"("error in (no error)"=w2960, "Interface in"=w2961) -> ("error out"=w2958:errorcluster, "output cluster"=w2957:T24, "Interface out"=w2962:refnum<class "Interface.lvclass">)  [unwired: 7 in]
                n1316 = Bundle By Name(cluster=w2957, "TRIGGER_MODE"=w2945) -> (w2959:T24)
                n1317 = call-dynamic "Set CCD_Config.vi"("error in (no error)"=w2958, "input cluster"=w2959, "Interface in"=w2962) -> ("error out"=w2956:errorcluster, "Interface out"=w2963:refnum<class "Interface.lvclass">)  [unwired: 7 in]
                n1318 = Flatten To String(anything=w2959, error in (no error)=w2956) -> (data string=w2954:string, error out=w2955:errorcluster)  [unwired: 2 in, 1 out]
                n1319 = call "Write flatted cluster.vi"("error in (no error)"=w2955, "flatted cluster"=w2954, "Interface in"=w2963) -> ("error out"=w2965:errorcluster, "Interface out"=w2964:refnum<class "Interface.lvclass">)  [unwired: 7 in]
                n1320 = call-dynamic "Write Interface.vi"("error in (no error)"=w2965, "Interface.lvclass"=w2964, "Channel in"=w2950) -> ("error out"=w2971:errorcluster, "Channel out"=w2972:refnum<class "Channel.lvclass">)  [unwired: 7 in]
                n1321 = call "Write section_name.vi"("error in (no error)"=w2971, "section_name"="CCD_ACS3", "Channel in"=w2972) -> ("error out"=w2969:errorcluster, "Channel out"=w2975:refnum<class "Channel.lvclass">)  [unwired: 7 in]
                n1322 = call-dynamic "save config.vi"("error in (no error)"=w2969, "file config"="lastsaved.cfg", "Channel in"=w2975) -> ("error out"=w2970:errorcluster, "Channel out"=w2976:refnum<class "Channel.lvclass">)  [unwired: 7 in]
                n1323 = call-dynamic "Read State Machine.vi"("error in (no error)"=w2970, "Device in"=w2976) -> ("error out"=w2966:errorcluster, "State Machine.lvclass"=w2978:refnum<class "State Machine.lvclass">, "Device out"=w2977:refnum<class "Channel.lvclass">)  [unwired: 7 in]
                n1324 = call-dynamic "Write State.vi"("error in (no error)"=w2966, "State"=60, "State Machine in"=w2978) -> ("error out"=w2967:errorcluster, "State Machine out"=w2979:refnum<class "State Machine.lvclass">)  [unwired: 7 in]
                n1325 = call-dynamic "Write State Machine.vi"("error in (no error)"=w2967, "State Machine.lvclass"=w2979, "Device in"=w2977) -> ("error out"=w2981:errorcluster, "Device out"=w2980:refnum<class "Channel.lvclass">)  [unwired: 7 in]
                n1326 = call-dynamic "Write Channel.vi"("error in (no error)"=w2981, "Channel.lvclass"=w2980, "Acquisition in"=w2951) -> ("error out"=w2946:errorcluster, "Acquisition out"=w2947:refnum<class "Acquisition.lvclass">)  [unwired: 7 in]
              }
            }
            n1327 = case shown="True" w2882 {
              tunnel: w2884 -> [w2905 w2910]
              tunnel: w2883 -> [w2904 w2909]
              tunnel: [w2905 w2908] -> w2855
              tunnel: [w2904 w2907] -> w2854
              tunnel: w2848 -> [_ w2906]
              frame False {
              }
              frame True {
                # "nome do arquivo .cfg"
                # "seção no arquivo .cfg"
                n1328 = call-dynamic "Read Channel.vi"("error in (no error)"=w2909, "Acquisition in"=w2910) -> ("error out"=w2939:errorcluster, "Channel.lvclass"=w2940:refnum<class "Channel.lvclass">, "Acquisition out"=w2941:refnum<class "Acquisition.lvclass">)  [unwired: 7 in]
                n1329 = call-dynamic "Read Interface.vi"("error in (no error)"=w2939, "Channel in"=w2940) -> ("error out"=w2932:errorcluster, "Interface.lvclass"=w2931:refnum<class "Interface.lvclass">, "Channel out"=w2942:refnum<class "Channel.lvclass">)  [unwired: 7 in]
                n1330 = call-dynamic "Get CCD_Config.vi"("error in (no error)"=w2932, "Interface in"=w2931) -> ("error out"=w2934:errorcluster, "output cluster"=w2935:T24, "Interface out"=w2930:refnum<class "Interface.lvclass">)  [unwired: 7 in]
                n1331 = Bundle By Name(cluster=w2935, "TRIGGER_MODE"=w2906) -> (w2933:T24)
                n1332 = call-dynamic "Set CCD_Config.vi"("error in (no error)"=w2934, "input cluster"=w2933, "Interface in"=w2930) -> ("error out"=w2936:errorcluster, "Interface out"=w2929:refnum<class "Interface.lvclass">)  [unwired: 7 in]
                n1333 = Flatten To String(anything=w2933, error in (no error)=w2936) -> (data string=w2938:string, error out=w2937:errorcluster)  [unwired: 2 in, 1 out]
                n1334 = call "Write flatted cluster.vi"("error in (no error)"=w2937, "flatted cluster"=w2938, "Interface in"=w2929) -> ("error out"=w2927:errorcluster, "Interface out"=w2928:refnum<class "Interface.lvclass">)  [unwired: 7 in]
                n1335 = call-dynamic "Write Interface.vi"("error in (no error)"=w2927, "Interface.lvclass"=w2928, "Channel in"=w2942) -> ("error out"=w2921:errorcluster, "Channel out"=w2920:refnum<class "Channel.lvclass">)  [unwired: 7 in]
                n1336 = call "Write section_name.vi"("error in (no error)"=w2921, "section_name"="CCD_ACS4", "Channel in"=w2920) -> ("error out"=w2923:errorcluster, "Channel out"=w2917:refnum<class "Channel.lvclass">)  [unwired: 7 in]
                n1337 = call-dynamic "save config.vi"("error in (no error)"=w2923, "file config"="lastsaved.cfg", "Channel in"=w2917) -> ("error out"=w2922:errorcluster, "Channel out"=w2916:refnum<class "Channel.lvclass">)  [unwired: 7 in]
                n1338 = call-dynamic "Read State Machine.vi"("error in (no error)"=w2922, "Device in"=w2916) -> ("error out"=w2926:errorcluster, "State Machine.lvclass"=w2914:refnum<class "State Machine.lvclass">, "Device out"=w2915:refnum<class "Channel.lvclass">)  [unwired: 7 in]
                n1339 = call-dynamic "Write State.vi"("error in (no error)"=w2926, "State"=60, "State Machine in"=w2914) -> ("error out"=w2925:errorcluster, "State Machine out"=w2913:refnum<class "State Machine.lvclass">)  [unwired: 7 in]
                n1340 = call-dynamic "Write State Machine.vi"("error in (no error)"=w2925, "State Machine.lvclass"=w2913, "Device in"=w2915) -> ("error out"=w2911:errorcluster, "Device out"=w2912:refnum<class "Channel.lvclass">)  [unwired: 7 in]
                n1341 = call-dynamic "Write Channel.vi"("error in (no error)"=w2911, "Channel.lvclass"=w2912, "Acquisition in"=w2941) -> ("error out"=w2907:errorcluster, "Acquisition out"=w2908:refnum<class "Acquisition.lvclass">)  [unwired: 7 in]
              }
            }
            n1342 = case shown="True" w2888 {
              tunnel: w2890 -> [w2983 w2988]
              tunnel: w2889 -> [w2982 w2987]
              tunnel: [w2983 w2986] -> w2859
              tunnel: [w2982 w2985] -> w2858
              tunnel: w2848 -> [_ w2984]
              frame False {
              }
              frame True {
                # "nome do arquivo .cfg"
                # "seção no arquivo .cfg"
                n1343 = call-dynamic "Read Channel.vi"("error in (no error)"=w2987, "Acquisition in"=w2988) -> ("error out"=w2992:errorcluster, "Channel.lvclass"=w2991:refnum<class "Channel.lvclass">, "Acquisition out"=w2990:refnum<class "Acquisition.lvclass">)  [unwired: 7 in]
                n1344 = call-dynamic "Read Interface.vi"("error in (no error)"=w2992, "Channel in"=w2991) -> ("error out"=w2999:errorcluster, "Interface.lvclass"=w3000:refnum<class "Interface.lvclass">, "Channel out"=w2989:refnum<class "Channel.lvclass">)  [unwired: 7 in]
                n1345 = call-dynamic "Get CCD_Config.vi"("error in (no error)"=w2999, "Interface in"=w3000) -> ("error out"=w2997:errorcluster, "output cluster"=w2996:T24, "Interface out"=w3001:refnum<class "Interface.lvclass">)  [unwired: 7 in]
                n1346 = Bundle By Name(cluster=w2996, "TRIGGER_MODE"=w2984) -> (w2998:T24)
                n1347 = call-dynamic "Set CCD_Config.vi"("error in (no error)"=w2997, "input cluster"=w2998, "Interface in"=w3001) -> ("error out"=w2995:errorcluster, "Interface out"=w3002:refnum<class "Interface.lvclass">)  [unwired: 7 in]
                n1348 = Flatten To String(anything=w2998, error in (no error)=w2995) -> (data string=w2993:string, error out=w2994:errorcluster)  [unwired: 2 in, 1 out]
                n1349 = call "Write flatted cluster.vi"("error in (no error)"=w2994, "flatted cluster"=w2993, "Interface in"=w3002) -> ("error out"=w3004:errorcluster, "Interface out"=w3003:refnum<class "Interface.lvclass">)  [unwired: 7 in]
                n1350 = call-dynamic "Write Interface.vi"("error in (no error)"=w3004, "Interface.lvclass"=w3003, "Channel in"=w2989) -> ("error out"=w3010:errorcluster, "Channel out"=w3011:refnum<class "Channel.lvclass">)  [unwired: 7 in]
                n1351 = call "Write section_name.vi"("error in (no error)"=w3010, "section_name"="CCD_ACS2", "Channel in"=w3011) -> ("error out"=w3008:errorcluster, "Channel out"=w3014:refnum<class "Channel.lvclass">)  [unwired: 7 in]
                n1352 = call-dynamic "save config.vi"("error in (no error)"=w3008, "file config"="lastsaved.cfg", "Channel in"=w3014) -> ("error out"=w3009:errorcluster, "Channel out"=w3015:refnum<class "Channel.lvclass">)  [unwired: 7 in]
                n1353 = call-dynamic "Read State Machine.vi"("error in (no error)"=w3009, "Device in"=w3015) -> ("error out"=w3005:errorcluster, "State Machine.lvclass"=w3017:refnum<class "State Machine.lvclass">, "Device out"=w3016:refnum<class "Channel.lvclass">)  [unwired: 7 in]
                n1354 = call-dynamic "Write State.vi"("error in (no error)"=w3005, "State"=60, "State Machine in"=w3017) -> ("error out"=w3006:errorcluster, "State Machine out"=w3018:refnum<class "State Machine.lvclass">)  [unwired: 7 in]
                n1355 = call-dynamic "Write State Machine.vi"("error in (no error)"=w3006, "State Machine.lvclass"=w3018, "Device in"=w3016) -> ("error out"=w3020:errorcluster, "Device out"=w3019:refnum<class "Channel.lvclass">)  [unwired: 7 in]
                n1356 = call-dynamic "Write Channel.vi"("error in (no error)"=w3020, "Channel.lvclass"=w3019, "Acquisition in"=w2990) -> ("error out"=w2985:errorcluster, "Acquisition out"=w2986:refnum<class "Acquisition.lvclass">)  [unwired: 7 in]
              }
            }
            n1357 = case shown="True" w2891 {
              tunnel: [w3021 w3055] -> w2860
              tunnel: [w3022 w3054] -> w2861
              tunnel: w2893 -> [w3022 w3025]
              tunnel: w2892 -> [w3021 w3024]
              tunnel: w2848 -> [_ w3023]
              frame False {
              }
              frame True {
                # "nome do arquivo .cfg"
                # "seção no arquivo .cfg"
                n1358 = call-dynamic "Read Channel.vi"("error in (no error)"=w3024, "Acquisition in"=w3025) -> ("error out"=w3056:errorcluster, "Channel.lvclass"=w3057:refnum<class "Channel.lvclass">, "Acquisition out"=w3058:refnum<class "Acquisition.lvclass">)  [unwired: 7 in]
